vi "validateIntegrationTime.vi"(11 "integrationTime":i32) -> (3 "validIntegrationTime":i32)   [LabVIEW 2015]
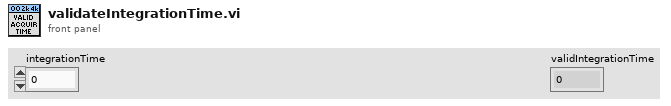
[diagram p1: front panel]
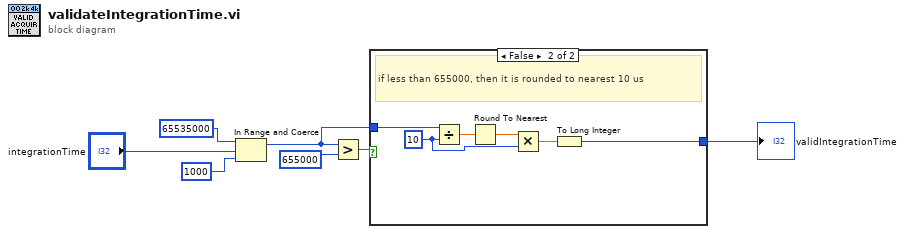
[diagram p0: block diagram]
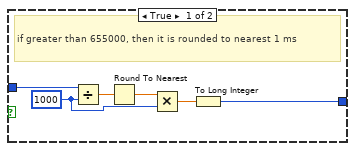
[diagram p2: hidden frame]
diagram:
  n1 = In Range and Coerce(upper limit=65535000, x="integrationTime", lower limit=1000) -> (coerced(x)=w2:i32)  [unwired: 1 out]
  n2 = Greater?(x=w2, y=655000) -> (0:w3:bool)
  n3 = case shown="False" w3 {
    tunnel: w2 -> [w13 w19]
    tunnel: [w8 w14] -> w1
    frame True {
      w12 = 1000 ("y")
      # "if greater than 655000, then it is rounded to nearest 1 ms"
      n4 = Divide(x=w13, y=w12) -> (x/y=w11:dbl)
      n5 = Round To Nearest(number=w11) -> (nearest integer value=w10:dbl)
      n6 = Multiply(x=w10, y=w12) -> (x*y=w9:dbl)
      n7 = To Long Integer(number=w9) -> (32bit integer=w8:i32)
    }
    frame False {
      w18 = 10 ("y")
      # "if less than 655000, then it is rounded to nearest 10 us"
      n8 = Divide(x=w19, y=w18) -> (x/y=w17:dbl)
      n9 = Round To Nearest(number=w17) -> (nearest integer value=w16:dbl)
      n10 = Multiply(x=w16, y=w18) -> (x*y=w15:dbl)
      n11 = To Long Integer(number=w15) -> (32bit integer=w14:i32)
    }
  }
  "validIntegrationTime" <- w1
